vi "CJ Theta (SubVI).vi"(0 "jav rad":dbl[](array[numeric])=[0.2, 0.2, 0.5], 1 "Brake":bool, 2 "error in":errorcluster, 3 "p_new":dbl[](array[numeric])=[2.0, 2.0, 0.0], 5 "Eta":dbl[](array[numeric])=[0.0, 0.0, 5.0, 0.0, 0.0, 0.0], 6 "Go":bool, 7 "p_old":dbl[](array[numeric])=[0.0, 0.0, 0.0], 11 "time":dbl) -> (8 "Arrived":bool, 12 "j":dbl, 13 "Theta_ddot":dbl[](array[numeric]), 14 "a":dbl, 15 "v":dbl, 16 "error out":errorcluster, 17 "p":dbl, 18 "Theta_d":dbl[](array[numeric]), 19 "omega":dbl[](array[numeric]))   [LabVIEW 2014]
uses:
  Library/Helping Routines/get_set_point_vec (SubVI).vi
  <vilib>/imath/engines/lvmath2/RunTimeEngine/ArithmeticOperatorToken/NIMS_ArithmeticOperator_multmx(M,CV).vi
  <instcachedir>/0/NIMS_ArithmeticOperator_multmx(M,CV)_787B4652E60B4C52835A7FB23671E425.lvgen/NIMS_ArithmeticOperator_multmx(M,CV)_787B4652E60B4C52835A7FB23671E425_000.vi
  <vilib>/imathl/engines/lvmath/Functions/Error Handling/Create Error.vi
  <vilib>/imath/engines/lvmath2/RunTimeEngine/NodeEndStatement/NIMS_NodeEndStatement_Get Vector.vi
  <instcachedir>/0/NIMS_NodeEndStatement_Get Vector_00D1625602D843AD9D7EC134A9EC13A2.lvgen/NIMS_NodeEndStatement_Get Vector_00D1625602D843AD9D7EC134A9EC13A2_001.vi
  <vilib>/imath/engines/lvmath2/RunTimeEngine/NodeEndStatement/NIMS_NodeEndStatement_Output.vi
  <instcachedir>/0/NIMS_NodeEndStatement_Output_53EC0D466D134D7ABD903AC30B43404B.lvgen/NIMS_NodeEndStatement_Output_53EC0D466D134D7ABD903AC30B43404B_005.vi
  <vilib>/imath/engines/lvmath2/RunTimeEngine/ErrorHandling/NIMS_Finalize Error.vi
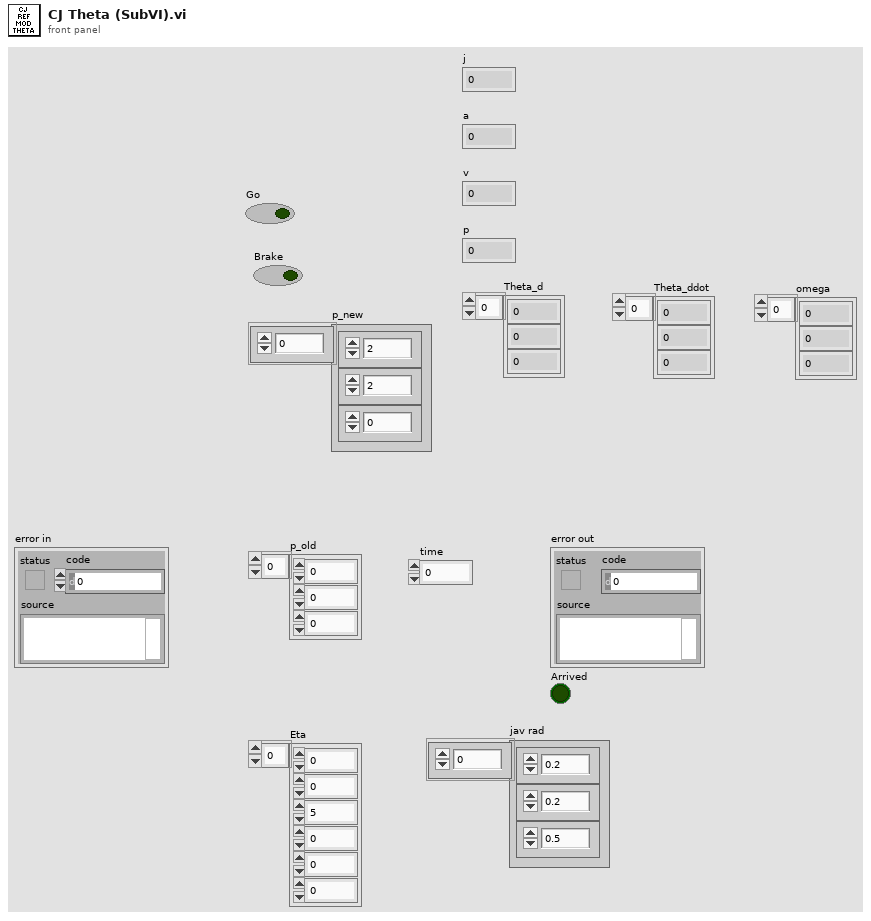
[diagram p1: front panel]
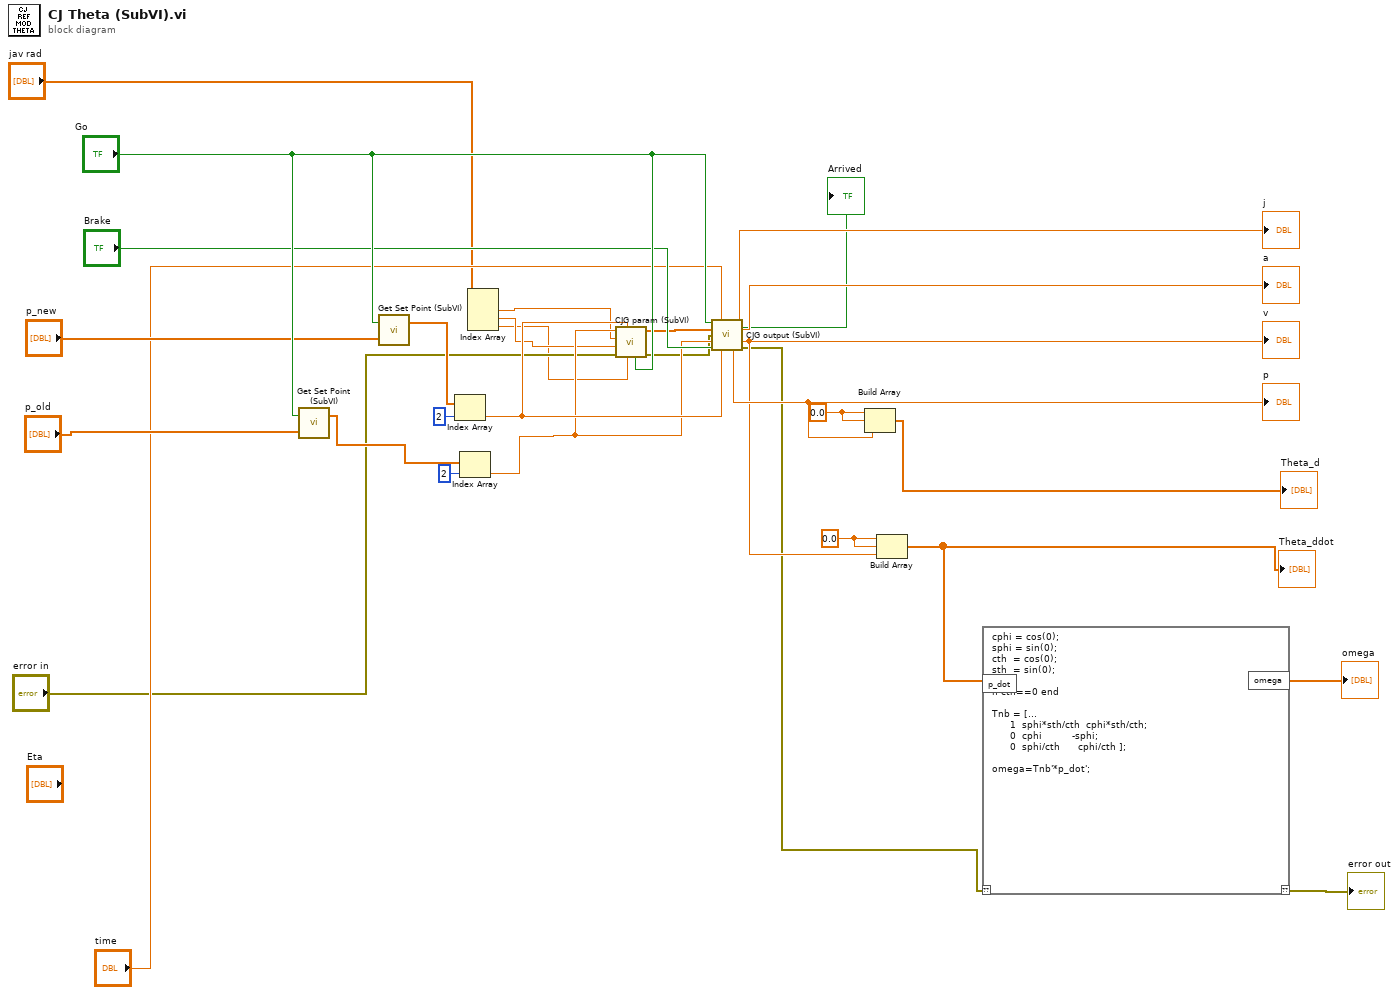
[diagram p0: block diagram]
diagram:
  w14 = 0.0 ("element")
  w16 = 0.0 ("element")
  n1 = call-poly "Get Set Point (SubVI).vi"("Set point in"="p_old", "auto set  in"="Go") -> ("Set point"=w18:dbl[])  [unwired: 1 out]
  n2 = call-poly "Get Set Point (SubVI).vi"("Set point in"="p_new", "auto set  in"="Go") -> ("Set point"=w22:dbl[])  [unwired: 1 out]
  n3 = Index Array(array=w22, index=2) -> (element=w20:dbl)
  n4 = Index Array(array=w18, index=2) -> (element=w17:dbl)
  n5 = Index Array(array="jav rad") -> (element #1=w3:dbl, element #2=w2:dbl, element #3=w1:dbl)  [unwired: 3 in]
  n6 = call "CJG param (SubVI).vi"("Boolean"="Go", "v_m"=w1, "p_m"=w20, "error in"="error in", "a_m"=w2, "j_m"=w3, "p_0"=w17) -> ("error out"=w8:errorcluster, "Array"=w23:dbl[])  [unwired: 3 in]
  n7 = call "CJG output (SubVI).vi"("Update"="Go", "time"="time", "parameters"=w23, "error in"=w8, "p_0"=w17, "Brake"="Brake", "p_m"=w20) -> ("Arrived"=→"Arrived":bool, "j"=→"j":dbl, "a"=→"a":dbl, "v"=w13:dbl, "p"=w15:dbl, "error out"=w7:errorcluster)  [unwired: 3 in]
  "p" <- w15
  "v" <- w13
  n8 = Build Array(w16, w16, w15) -> (→"Theta_d":dbl[])
  n9 = Build Array(w14, w14, w13) -> (w11:dbl[])
  "Theta_ddot" <- w11
  n10 = mathscript code="cphi = cos(0);\nsphi = sin(0);\ncth  = cos(0);\nsth  = sin(0);\n  \nif cth==0 end\n \nTnb = [...\n      1  sphi*sth/cth  cphi*sth/cth;\n      0  cphi          -sphi;\n      0  sphi/cth      cphi/cth ];\n\nomega=Tnb'*p_dot';"("??"=w7, "p_dot"=w11) -> ("??"=→"error out":errorcluster, "omega"=→"omega":dbl[])
